vi "Build Parameter.vi"(7 "Return Parameter? (T)":bool=TRUE, 10 "Value":string, 11 "Key":string) -> (3 "Parameter Array":T1[](array[typedef]))   [LabVIEW 2011, in "i3-oauth.lvlib"]
doc: "Used to help create the Parameter Arrays (URL, Header, and Body parameter arrays) used by the Authenticate with Access Token VI for creating the OAuth signature. Use the <b>Parameter Array</b> output with a Build Array configured for concatenation to package multiple parameters together.\n\n<b>Advanced Usage:</b>\nParameters can be conditionally added by changing the value of <b>Return Parameter?</b>. If Return Parameter? is true then a <b>Name-Value Pair</b> array with a single element is returned that represents the input <b>Key</b> and <b>Value</b>. If Return Parameter? is false then an empty <b>Name-Value Pair</b> array is returned that will cause no modification when used with Build Array."
uses:
  i3-oauth.lvlib
  Controls/Name-Value Pair.ctl
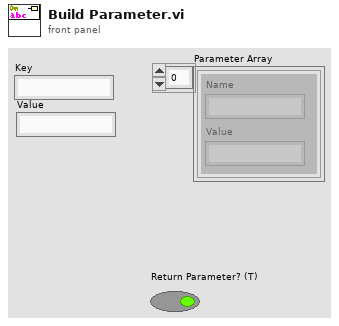
[diagram p1: front panel]
types:
  T1 = typedef "i3-oauth.lvlib/Name-Value Pair.ctl" = cluster{"Name":string, "Value":string}
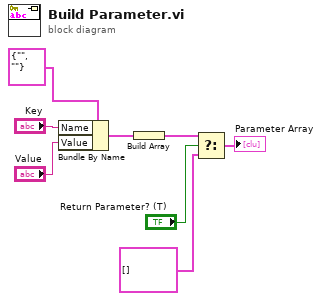
[diagram p0: block diagram]
diagram:
  n1 = Bundle By Name(cluster=T1 {"Name"="", "Value"=""} ("pair"), "Name"="Key", "Value"="Value") -> (w7:T1)
  n2 = Build Array(w7) -> (w4:T1[])
  n3 = Select(t=w4, s="Return Parameter? (T)", f=T1[] [] ("appended array")) -> (s? t:f=→"Parameter Array":T1[])
